vi "RTM - Apply Rx Configuration.vi"(8 "error in (no error)":errorcluster, 11 "Node Ptr":T1 format="%.0x") -> (0 "error out":errorcluster)   [LabVIEW 2019, in "UDP-Custom-Device System Explorer.lvlib"]
uses:
  UDP-Custom-Device System Explorer.lvlib
  <vilib>/NI VeriStand/Custom Device API/Custom Device Item Ref.ctl
  <vilib>/NI VeriStand/Custom Device API/Custom Device Channel.ctl
  <vilib>/NI VeriStand/Custom Device API/Custom Device Channel Type.ctl
  Shared/Constants.vi
  <vilib>/NI VeriStand/Custom Device API/Custom Device API.lvlib
  Property Accessors/Shared Channel Accessors.lvlib
  Shared/UDP-Custom-Device Shared.lvlib
  Property Accessors/Rx Channel Accessors.lvlib
  Property Accessors/Rx Channel Section Accessors.lvlib
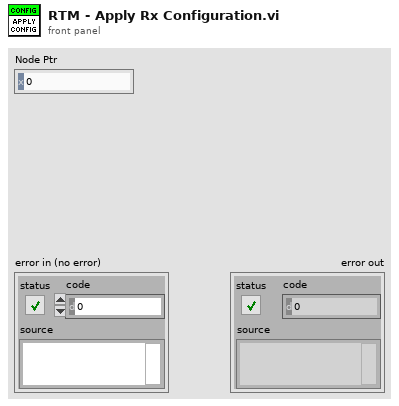
[diagram p1: front panel]
types:
  T1 = typedef "Custom Device API.lvlib/Custom Device Item Ref.ctl" = u64
  T2 = typedef "Custom Device API.lvlib/Custom Device Channel.ctl" = cluster{"Type":T3, "Units":string, "Default Value":dbl, "Faultable":bool, "Scalable":bool}
  T3 = typedef "Custom Device API.lvlib/Custom Device Channel Type.ctl" = enum16{"Input", "Output"}
  T4 = typedef "UDP-Custom-Device Shared.lvlib/Shared - Channel Data Type.ctl" = enum16{"Boolean", "Single", "Double", "I8", "I16", "I32", "I64", "U8", "U16", "U32", "U64"}
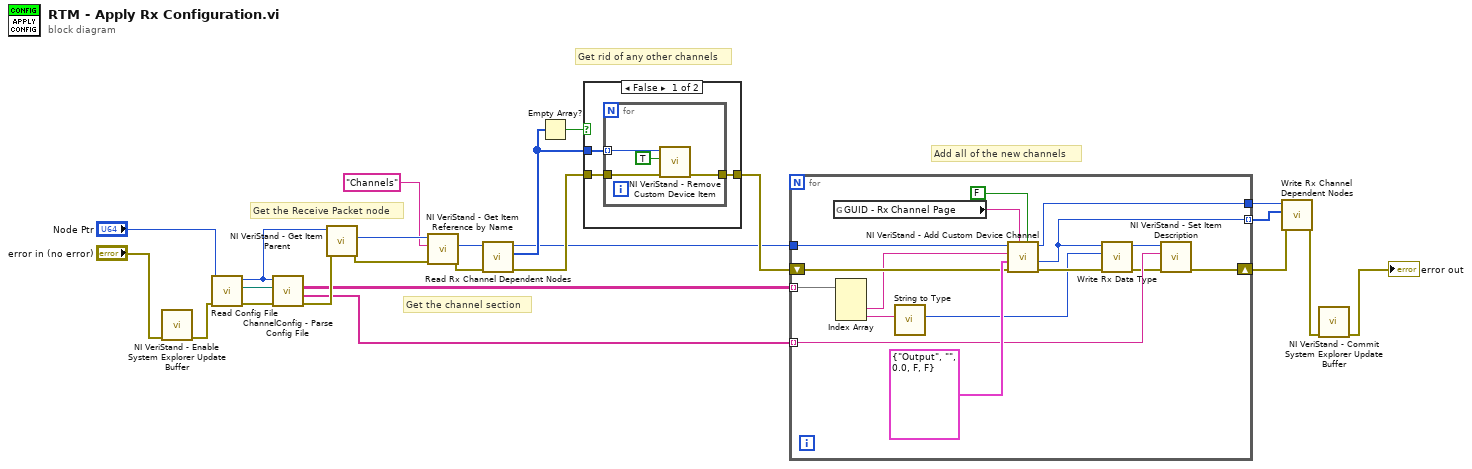
[diagram p0: block diagram]
diagram:
  # "Get the channel section"
  # "Add all of the new channels"
  # "Get rid of any other channels"
  # "Get the Receive Packet node"
  n1 = call <vilib>:"NI VeriStand - Enable System Explorer Update Buffer.vi"("error in (no error)"="error in (no error)") -> ("error out"=w14:errorcluster)  [unwired: 10 in]
  n2 = call "Read Config File.vi"("error in (no error)"=w14, "Node Ptr"="Node Ptr") -> ("error out"=w23:errorcluster, "Config File"=w22:path, "Node Ptr out"=w24:T1)  [unwired: 7 in]
  n3 = call "ChannelConfig - Parse Config File.vi"("error in (no error)"=w23, "Config Path"=w22, "Node Ptr"=w24) -> ("error out"=w21:errorcluster, "Descriptions"=w19:string[], "Channel Configuration"=w20:string[][])  [unwired: 6 in]
  n4 = call <vilib>:"NI VeriStand - Get Item Parent.vi"("error in (no error)"=w21, "Item Ref in"=w24) -> ("error out"=w11:errorcluster, "Parent Ref"=w12:T1)  [unwired: 6 in, 2 out]
  n5 = call <vilib>:"NI VeriStand - Get Item Reference by Name.vi"("error in (no error)"=w11, "Item Name"="Channels" ("Section Name"), "Parent Ref in"=w12) -> ("error out"=w4:errorcluster, "Item Ref"=w5:T1)  [unwired: 5 in, 2 out]
  n6 = call "Read Rx Channel Dependent Nodes.vi"("error in (no error)"=w4, "Node Ptr"=w5) -> ("error out"=w3:errorcluster, "Dependent Node Refs"=w2:T1[], "Node Ptr out"=w1:T1)  [unwired: 7 in]
  n7 = Empty Array?(array=w2) -> (empty?=w17:bool)
  n8 = case shown="False" w17 {
    tunnel: [w27 w32] -> w18
    tunnel: w3 -> [w26 w32]
    tunnel: w2 -> [w25 _]
    frame False {
      n9 = for {
        tunnel: w25 -> [w31] mode=indexing
        tunnel: [w29] -> w27
        tunnel: w26 -> [w28]
        n10 = call <vilib>:"NI VeriStand - Remove Custom Device Item.vi"("error in (no error)"=w28, "Force Delete (F)"=TRUE, "Item Ref in"=w31) -> ("error out"=w29:errorcluster)  [unwired: 7 in, 1 out]
      }
    }
    frame True {
    }
  }
  n11 = for {
    tunnel: w1 -> [w45]
    tunnel: w20 -> [w40] mode=indexing
    tunnel: w19 -> [w38] mode=indexing
    shift-right: [w43] -> w7
    shift-left: w18 -> [w41]
    tunnel: [w34] -> w8 mode=indexing
    tunnel: [w33] -> w9
    n12 = global read "Constants.vi" "GUID - Rx Channel Page"() -> (w46:string)
    n13 = Index Array(array=w40) -> (element #2=w39:string, element #3=w36:string)  [unwired: 3 in, 1 out]
    n14 = call "String to Type.vi"("String Type"=w36) -> ("Data Type"=w35:T4)  [unwired: 10 in]
    n15 = call <vilib>:"NI VeriStand - Add Custom Device Channel.vi"("Highlight? (F)"=FALSE, "GUID (Default Channel)"=w46, "error in (no error)"=w41, "Channel"=T2 {"Type"=enum."Output", "Units"="", "Default Value"=0.0, "Faultable"=FALSE, "Scalable"=FALSE}, "Channel Name"=w39, "Parent Ref in"=w45) -> ("error out"=w48:errorcluster, "Channel Ref"=w34:T1, "Parent Ref out"=w33:T1)  [unwired: 2 in, 1 out]
    n16 = call "Write Rx Data Type.vi"("error in (no error)"=w48, "Data Type"=w35, "Node Ptr"=w34) -> ("error out"=w37:errorcluster, "Node Ptr out"=w42:T1)  [unwired: 7 in]
    n17 = call <vilib>:"NI VeriStand - Set Item Description.vi"("error in (no error)"=w37, "Description"=w38, "Item Ref in"=w42) -> ("error out"=w43:errorcluster)  [unwired: 6 in, 2 out]
  }
  n18 = call "Write Rx Channel Dependent Nodes.vi"("error in (no error)"=w7, "Dependent Node Refs"=w8, "Node Ptr"=w9) -> ("error out"=w6:errorcluster)  [unwired: 7 in, 1 out]
  n19 = call <vilib>:"NI VeriStand - Commit System Explorer Update Buffer.vi"("error in (no error)"=w6) -> ("error out"=→"error out":errorcluster)  [unwired: 10 in]
